vi "Item List_Write.vi"(4 "error in (no error)":errorcluster, 5 "Value":string[](array[string]), 6 "Container State":T2, 7 "Display State In":T1) -> (0 "error out":errorcluster, 3 "Display State Out":T1)   [LabVIEW 2010, in "magic ring.xctl"]
uses:
  magic ring.xctl
  <vilib>/_xctls/Container State.ctl
  controls/State.ctl
  <vilib>/_xctls/XControlSupport.lvlib
panel:
  # "Replace the Value Control below with a Control of desired type.\nDo not remove this Control or the others from the connector pane.\nDo not change the connector pane pattern.\nThe Value control should always be the third terminal from top on the input side in the connector pane."
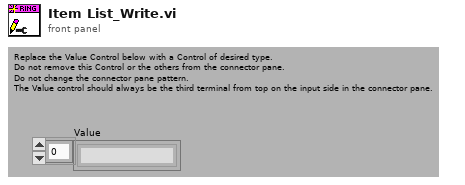
[diagram p1: front panel]
types:
  T1 = typedef "magic ring.xctl/State.ctl" = cluster{"item list":string[], "displayed items":string[], "max rows (5)":i32, "min rows (2)":i32, "selection":i32}
  T2 = typedef "XControlSupport.lvlib/Container State.ctl" = cluster{"Indicator?":bool, "Run Mode?":bool, " Refnum":refnum<vi>}
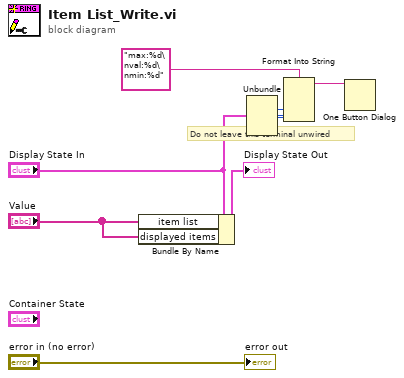
[diagram p0: block diagram]
diagram:
  # "Do not leave this terminal unwired"
  n1 = Bundle By Name(cluster="Display State In", "item list"="Value", "displayed items"="Value") -> (→"Display State Out":T1)
  n2 = Unbundle("Display State In") -> ("max rows (5)"=w5:i32, "min rows (2)"=w4:i32, "selection"=w3:i32)  [unwired: 2 out]
  n3 = Format Into String(format string="max:%d\nval:%d\nmin:%d", w5, w3, w4) -> (resulting string=w7:string)  [unwired: 2 in, 1 out]
  n4 = One Button Dialog(message=w7) -> ()  [unwired: 1 in, 1 out]
  "error out" <- "error in (no error)"
